vi "assembleScanInfo.vi"(6 "volume info":T1, 7 "center of mass":T2, 9 "current location":T2, 10 "message":T4(ring), 11 "scan info":T3) -> (3 "scan info out":T3)   [LabVIEW 2010]
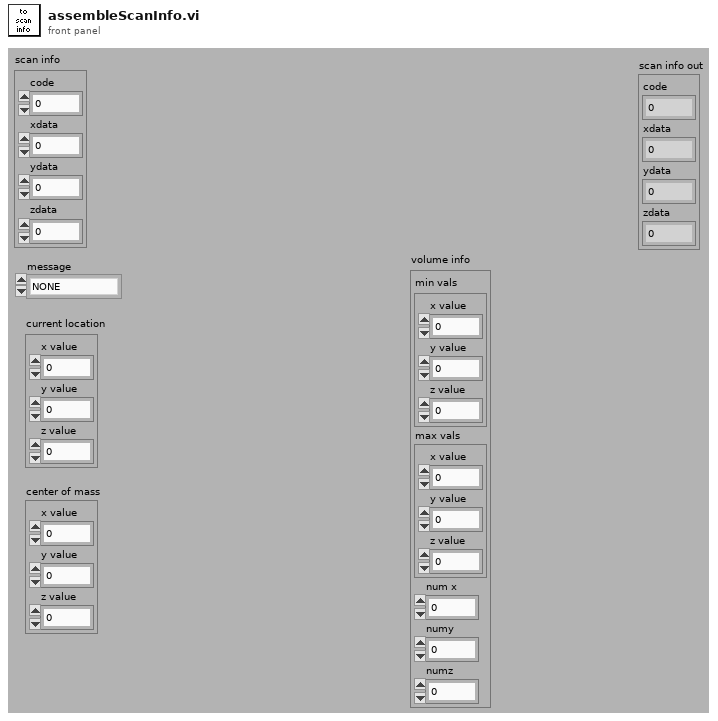
[diagram p1: front panel]
types:
  T1 = cluster{"min vals":cluster{"x value":i16, "y value":i16, "z value":i16}, "max vals":cluster{"x value":i16, "y value":i16, "z value":i16}, "num x":u32, "numy":u32, "numz":u32}
  T2 = cluster{"x value":i16, "y value":i16, "z value":i16}
  T3 = cluster{"code":i32, "xdata":i32, "ydata":i32, "zdata":i32}
  T4 = enum16{"NONE", "VOLUME_START", "LINE_START", "LINE_END", "VOLUME_END"}
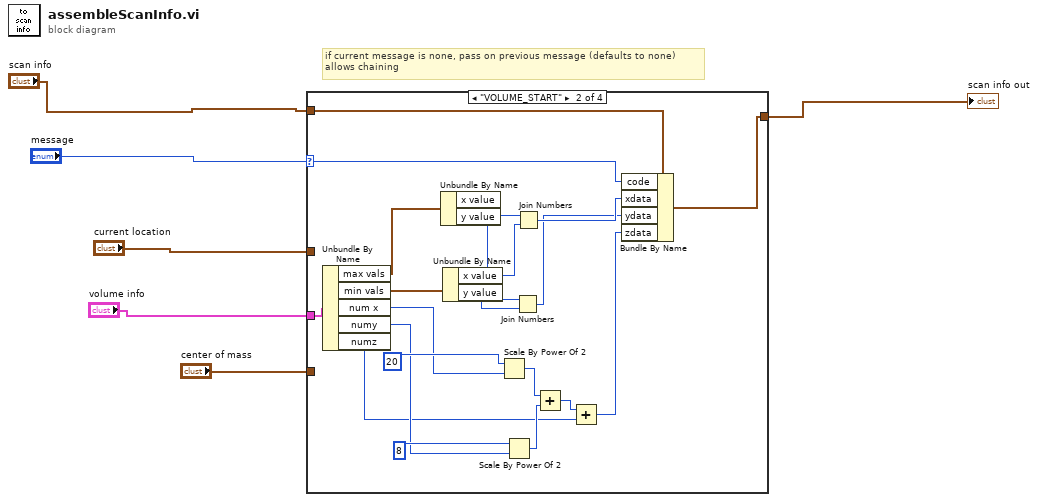
[diagram p0: block diagram]
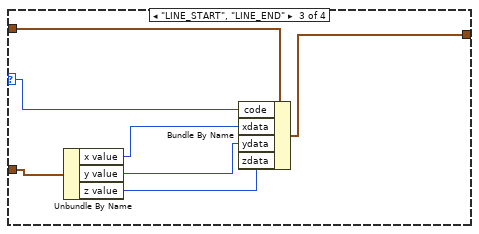
[diagram p3: hidden frame]
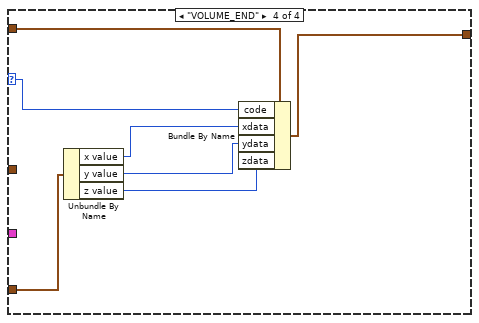
[diagram p4: hidden frame]
diagram:
  # "if current message is none, pass on previous message (defaults to none)\nallows chaining"
  n1 = case shown="\"VOLUME_START\"" "message" {
    selector: "message" -> [_ w18 w35 w42]
    tunnel: "scan info" -> [w7 w19 w30 w38]
    tunnel: [w7 w14 w31 w39] -> w4
    tunnel: "current location" -> [_ _ w34 _]
    tunnel: "center of mass" -> [_ _ _ w36]
    tunnel: "volume info" -> [_ w13 _ _]
    frame "NONE", Default {
    }
    frame "VOLUME_START" {
      n2 = Unbundle By Name(w13) -> ("max vals"=w12:T2, "min vals"=w11:T2, "num x"=w10:u32, "numy"=w9:u32, "numz"=w8:u32)
      n3 = Unbundle By Name(w12) -> ("x value"=w28:i16, "y value"=w26:i16)
      n4 = Unbundle By Name(w11) -> ("x value"=w27:i16, "y value"=w25:i16)
      n5 = Scale By Power Of 2(n=u8 20 ("x"), x=w10) -> (x*2^n=w24:u32)
      n6 = Scale By Power Of 2(n=u8 8 ("x"), x=w9) -> (x*2^n=w21:u32)
      n7 = Join Numbers(hi=w26, lo=w25) -> ((hi.lo)=w16:u32)
      n8 = Join Numbers(hi=w28, lo=w27) -> ((hi.lo)=w17:u32)
      n9 = Add(x=w24, y=w21) -> (x+y=w20:u32)
      n10 = Add(x=w20, y=w8) -> (x+y=w15:u32)
      n11 = Bundle By Name(cluster=w19, "code"=w18, "xdata"=w17, "ydata"=w16, "zdata"=w15) -> (w14:T3)
    }
    frame "LINE_START", "LINE_END" {
      n12 = Unbundle By Name(w34) -> ("x value"=w33:i16, "y value"=w32:i16, "z value"=w29:i16)
      n13 = Bundle By Name(cluster=w30, "code"=w35, "xdata"=w33, "ydata"=w32, "zdata"=w29) -> (w31:T3)
    }
    frame "VOLUME_END" {
      n14 = Unbundle By Name(w36) -> ("x value"=w41:i16, "y value"=w40:i16, "z value"=w37:i16)
      n15 = Bundle By Name(cluster=w38, "code"=w42, "xdata"=w41, "ydata"=w40, "zdata"=w37) -> (w39:T3)
    }
  }
  "scan info out" <- w4
